vi "Pfeiffer-RVC300.set pressure.vi"(0 "i ref in":refnum<vi>, 1 "pressure":dbl, 3 "ms timeout (10000)":i32=10000, 5 "error in (no error)":errorcluster) -> (14 "i ref out":refnum<vi>, 17 "timed out":bool, 19 "error out":errorcluster)   [LabVIEW 2014, in "Pfeiffer-RVC300.lvlib"]
doc: "Sets the pressure for pressure regulation.\n\nLicense Agreement for this software:\n\nCopyright (C)\nMax-Planck-Institut für Kernphysik\nSaupfercheckweg 1\n69117 Heidelberg\nGermany\n\nContact: christopher.borgmann@mpi-hd.mpg.de\n\nThis program is free software: you can redistribute it and/or modify \nit under the terms of the GNU General Public License as published by\nthe Free Software Foundation, either version 3 of the License, or\n(at your option) any later version.\n\nThis program is distributed in the hope that it will be useful,\nbut WITHOUT ANY WARRANTY; without even the implied warranty of\nMERCHANTABILITY or FITNESS FOR A PARTICULAR PURPOSE. See the\nGNU General Public License for more details.\n\nYou should have received a copy of the GNU General Public License\nalong with this program. If not, see <http://www.gnu.org/licenses/>.\n\nMax-Planck-Institut für Kernphysik\nSaupfercheckweg 1, 69117 Heidelberg, Germany\nFor all questions and ideas contact: christopher.borgmann@mpi-hd.mpg.de\nLast update: 08.07.2010"
uses:
  Pfeiffer-RVC300.lvlib
  CSCore/CSApplicationBaseClasses/DeviceBase/DeviceBase.lvlib
  CSlibraries-extern/DimLVEvent/LVDimInterface/LVDimInterface.lvlib
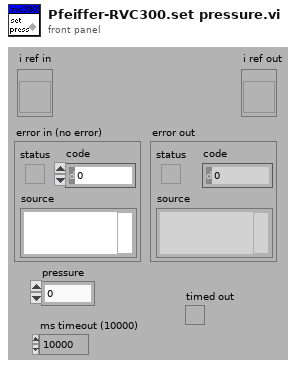
[diagram p1: front panel]
types:
  T1 = typedef "Pfeiffer-RVC300.lvlib/Pfeiffer-RVC300.i attribute.ctl" = cluster{"interfaceInitialized":bool, "VISAResource":refnum<visa-resource-name>, "WaitingTime":u32, "nomValues":T2, "actValues":T2}
  T2 = typedef "Pfeiffer-RVC300.lvlib/Pfeiffer-RVC300.parameters.ctl" = cluster{"regulationMode":T3, "valveType":string, "sensorType":string, "valveState":string, "flow":dbl, "pressure":dbl, "serviceIDs":cluster{"regulationModeID":i32, "valveTypeID":i32, "sensorTypeID":i32, "valveStateID":i32, "flowID":i32, "pressureID":i32}}
  T3 = typedef "Pfeiffer-RVC300.lvlib/Pfeiffer-RVC300.regulation mode.ctl" = enum16{"unknown", "Pressure", "Flow", "Wait"}
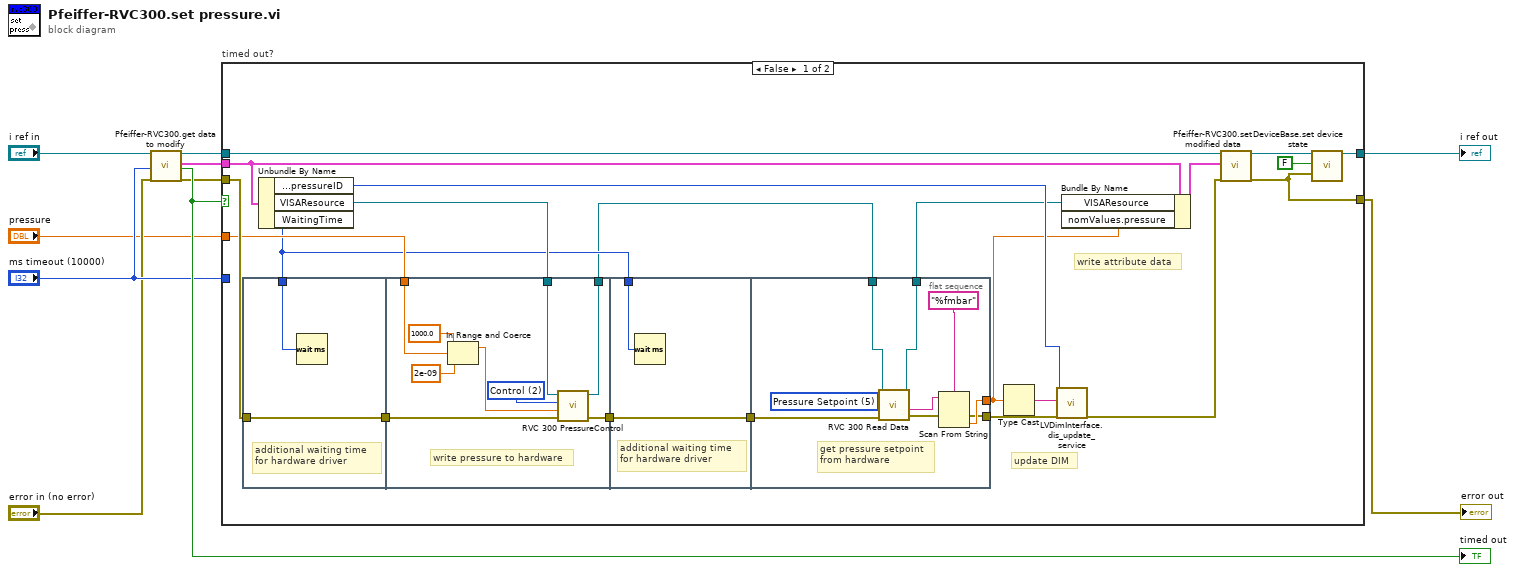
[diagram p0: block diagram]
diagram:
  n1 = call "Pfeiffer-RVC300.get data to modify.vi"("i ref in"="i ref in", "ms timeout (10000)"="ms timeout (10000)", "error in (no error)"="error in (no error)") -> ("i ref out"=w4:refnum<vi>, "i attribute"=w2:T1, "timed out"=w7:bool, "error out"=w3:errorcluster)  [unwired: 13 in]
  "timed out" <- w7
  n2 = case "timed out?" shown="False" w7 {
    tunnel: [w28 w55] -> w9
    tunnel: w4 -> [w31 w55]
    tunnel: [w26 w54] -> w8
    tunnel: w3 -> [w25 w54]
    tunnel: w2 -> [w23 _]
    tunnel: "ms timeout (10000)" -> [_ _]
    tunnel: "pressure" -> [w17 _]
    frame False {
      # "write attribute data"
      # "update DIM"
      n3 = flat-sequence {
        tunnel: w25 -> [w33]
        tunnel: [w33] -> w24
        tunnel: w15 -> [w32]
        tunnel: w24 -> [w42]
        tunnel: w22 -> [w39]
        tunnel: [w40] -> w13
        tunnel: w17 -> [w36]
        tunnel: [w41] -> w16
        tunnel: w16 -> [w44]
        tunnel: w15 -> [w43]
        tunnel: [w44] -> w14
        tunnel: [w45] -> w18
        tunnel: w14 -> [w53]
        tunnel: w13 -> [w52]
        tunnel: [w51] -> w12
        tunnel: [w48] -> w11
        frame #0 {
          # "additional waiting time \nfor hardware driver"
          n4 = Wait (ms)(milliseconds to wait=w32) -> ()  [unwired: 1 out]
        }
        frame #1 {
          w38 = u16 2 items=["Close", "Open", "Control"] ("Action")
          # "write pressure to hardware"
          n5 = In Range and Coerce(upper limit=1000.0, x=w36, lower limit=2e-09) -> (coerced(x)=w37:dbl)  [unwired: 1 out]
          n6 = call "RVC 300 PressureControl.vi"("error in"=w42, "Pressure"=w37, "Action"=w38, "Resource Name"=w39) -> ("error out"=w41:errorcluster, "Resource Name out"=w40:refnum<visa-resource-name>)  [unwired: 2 in]
        }
        frame #2 {
          # "additional waiting time \nfor hardware driver"
          n7 = Wait (ms)(milliseconds to wait=w43) -> ()  [unwired: 1 out]
        }
        frame #3 {
          w50 = u16 5 items=["Mode", "Pressure", "Unit", "Firmwareversion", "Keyboard lock", "Pressure Setpoint", "Sensor Type", "Valve Type"] ("RVC 300 Read")
          # "get pressure setpoint \nfrom hardware"
          n8 = call "RVC 300 Read Data.vi"("error in"=w53, "RVC 300 Read"=w50, "Resource Name"=w52) -> ("error out"=w46:errorcluster, "Response Data out"=w47:string, "Resource Name out"=w51:refnum<visa-resource-name>)  [unwired: 5 in, 1 out]
          n9 = Scan From String(format string="%fmbar", input string=w47, error in=w46) -> (error out=w45:errorcluster, output 1=w48:dbl)  [unwired: 2 in, 2 out]
        }
      }
      n10 = Unbundle By Name(w23) -> ("nomValues.serviceIDs.pressureID"=w21:i32, "VISAResource"=w22:refnum<visa-resource-name>, "WaitingTime"=w15:u32)
      n11 = Type Cast(x=w11) -> (*(type *) &x=w20:string)  [unwired: 1 in]
      n12 = call "LVDimInterface.dis_update_service.vi"("my_serviceID"=w21, "data"=w20, "error in (no error)"=w18) -> ("error out"=w19:errorcluster)  [unwired: 14 in, 2 out]
      n13 = Bundle By Name(cluster=w23, "VISAResource"=w12, "nomValues.pressure"=w11) -> (w30:T1)
      n14 = call "Pfeiffer-RVC300.set modified data.vi"("i ref in"=w31, "i attribute"=w30, "error in (no error)"=w19) -> ("i ref out"=w29:refnum<vi>, "error out"=w26:errorcluster)  [unwired: 15 in]
      n15 = call "DeviceBase.set device state.vi"("i ref in"=w29, "implicit"=FALSE, "device error"=w26) -> ("i ref out"=w28:refnum<vi>)  [unwired: 14 in, 2 out]
    }
    frame True {
    }
  }
  "error out" <- w8
  "i ref out" <- w9
